vi "format status message v2 SmartMotor-Wrapper.vi"(8 "error in (no error)":errorcluster, 9 "status msg":string, 11 "Str Refnum":refnum<vi>) -> (0 "error out":errorcluster, 1 "Output String (this call)":string, 2 "Output String (aggregate)":string, 3 "Str Refnum out":refnum<vi>)   [LabVIEW 2020]
doc: "Developed by Kevin Thompson\nThompson Engineering, LLC\nkevin@thompsonengineering.net"
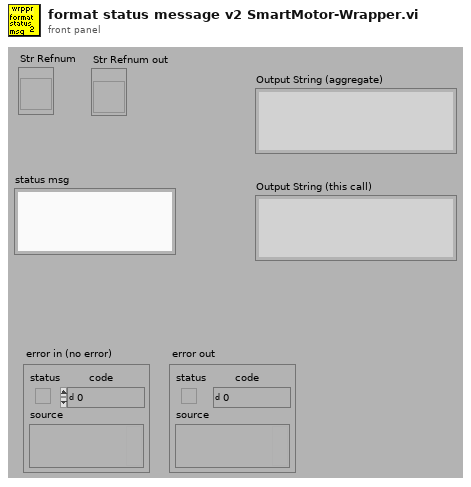
[diagram p1: front panel]
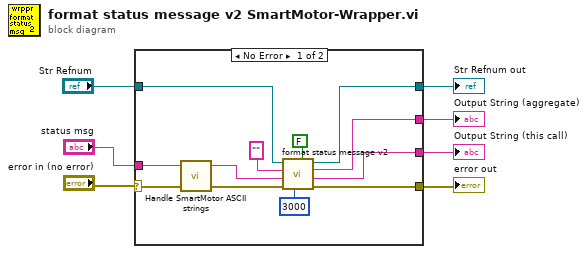
[diagram p0: block diagram]
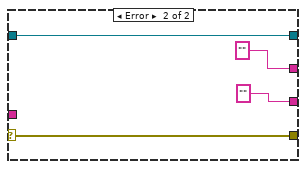
[diagram p2: hidden frame]
diagram:
  n1 = case shown="No Error" "error in (no error)" {
    selector: "error in (no error)" -> [w11 w22]
    tunnel: "Str Refnum" -> [w19 w23]
    tunnel: [w17 w22] -> w6
    tunnel: [w16 ""] -> w5
    tunnel: [w18 w23] -> w4
    tunnel: [w15 ""] -> w3
    tunnel: "status msg" -> [w8 _]
    frame No Error {
      n2 = call "Handle SmartMotor ASCII strings.vi"("error in (no error)"=w11, "String in"=w8) -> ("error out"=w10:errorcluster, "String out"=w9:string)  [unwired: 2 in]
      n3 = call <vilib>:"format status message v2.vi"("use marker? (T)"=FALSE, "max chars (2000)"=3000, "error in (no error)"=w10, "status msg"=w9, "Instance string"="", "Str Refnum"=w19) -> ("error out"=w17:errorcluster, "Output String (this call)"=w15:string, "Output String (aggregate)"=w16:string, "Str Refnum out"=w18:refnum<vi>)  [unwired: 1 in, 1 out]
    }
    frame Error {
    }
  }
  "error out" <- w6
  "Output String (this call)" <- w3
  "Output String (aggregate)" <- w5
  "Str Refnum out" <- w4
